vi "ziSelectDevice.vi"(3 "Error In":errorcluster, 4 "Device (first)":string, 5 "Handle In":T1 {"Handle" format="0x%08x"; "Conn" format="0x%08x"}) -> (0 "Error Out":errorcluster, 1 "Selected Device":string, 2 "Handle Out":T1 {"Handle" format="0x%08x"; "Conn" format="0x%08x"})   [LabVIEW 2016, in "Zurich Instruments LabOne.lvlib"]
doc: "Selects to the default device to use."
uses:
  Zurich Instruments LabOne.lvlib
  ziTypeHandle.ctl
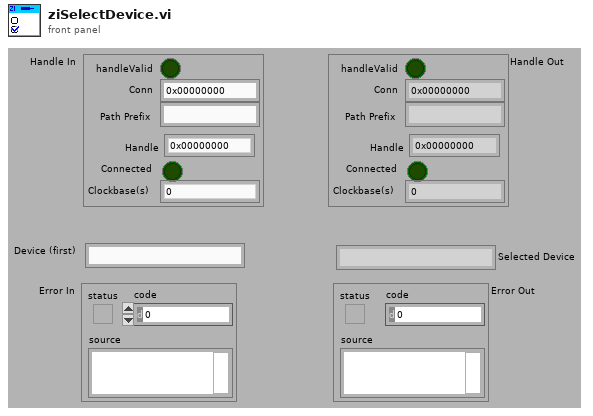
[diagram p1: front panel]
types:
  T1 = typedef "Zurich Instruments LabOne.lvlib/ziTypeHandle.ctl" = cluster{"handleValid":bool, "Conn":u64, "Path Prefix":string, "Handle":u64, "Connected":bool, "Clockbase(s)":dbl}
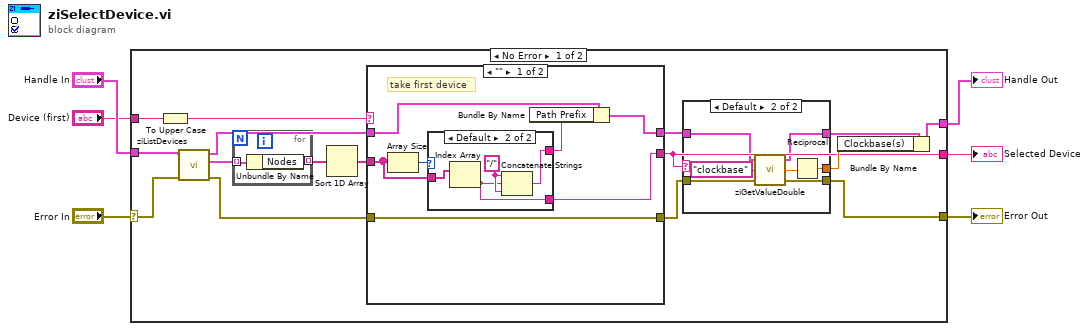
[diagram p0: block diagram]
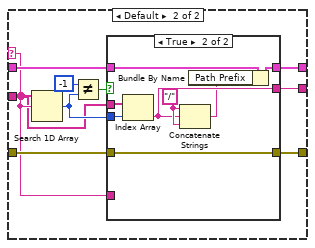
[diagram p4: hidden frame]
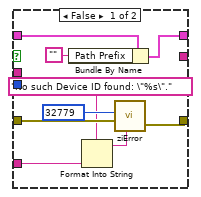
[diagram p5: hidden frame]
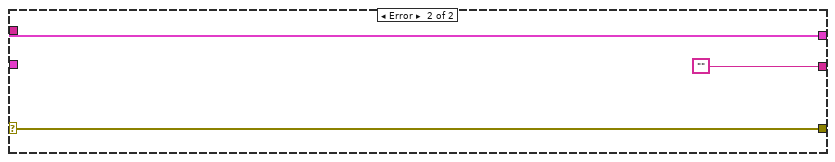
[diagram p6: hidden frame]
diagram:
  n1 = case shown="No Error" "Error In" {
    selector: "Error In" -> [w14 w72]
    tunnel: "Handle In" -> [w22 w74]
    tunnel: "Device (first)" -> [w21 _]
    tunnel: [w16 w74] -> w4
    tunnel: [w18 w72] -> w3
    tunnel: [w9 ""] -> w2
    frame No Error {
      n2 = To Upper Case(1:w21) -> (0:w13:string)
      n3 = call "ziListDevices.vi"("Error In"=w14, "Handle In"=w22) -> ("Error Out"=w12:errorcluster, "Devices"=w20:cluster{"Nodes":string, i32}[], "Handle Out"=w10:T1)  [unwired: 3 out]
      n4 = for {
        tunnel: w20 -> [w33] mode=indexing
        tunnel: [w32] -> w19 mode=indexing
        n5 = Unbundle By Name(w33) -> ("Nodes"=w32:string)
      }
      n6 = Sort 1D Array(array=w19) -> (sorted array=w7:string[])
      n7 = case shown="\"\"" w13 {
        selector: w13 -> [_ w50]
        tunnel: w7 -> [w35 w48]
        tunnel: w12 -> [w34 w51]
        tunnel: [w38 w53] -> w11
        tunnel: w10 -> [w39 w52]
        tunnel: [w36 w46] -> w9
        tunnel: [w34 w45] -> w8
        frame "" {
          # "take first device"
          n8 = Array Size(array=w35) -> (size(s)=w40:i32)
          n9 = case shown="Default" w40 {
            tunnel: [_ w43] -> w37
            tunnel: [_ w42] -> w36
            tunnel: w35 -> [_ w41]
            frame 0 {
              # "no device found"
            }
            frame Default {
              w44 = "/" ("string")
              n10 = Index Array(array=w41) -> (element=w42:string)  [unwired: 1 in]
              n11 = Concatenate Strings(w44, w42, w44) -> (w43:string)
            }
          }
          n12 = Bundle By Name(cluster=w39, "Path Prefix"=w37) -> (w38:T1)
        }
        frame Default {
          n13 = Search 1D Array(1D array=w48, element=w50) -> (index of element=w49:i32)  [unwired: 1 out]
          n14 = Not Equal?(x=-1, y=w49) -> (x != y?=w47:bool)
          n15 = case shown="True" w47 {
            tunnel: w49 -> [_ w70]
            tunnel: w48 -> [_ w71]
            tunnel: w52 -> [w63 w69]
            tunnel: [w62 w67] -> w53
            tunnel: [_ w66] -> w46
            tunnel: [w60 w64] -> w45
            tunnel: w51 -> [w61 w64]
            tunnel: w50 -> [w57 _]
            frame False {
              n16 = Bundle By Name(cluster=w63, "Path Prefix"="") -> (w62:T1)
              n17 = Format Into String(format string="No such Device ID found: \"%s\"." ("source"), w57) -> (resulting string=w56:string)  [unwired: 2 in, 1 out]
              n18 = call "ziError.vi"("ziErrorCode"=u32 32779, "Error In"=w61, "Annotation"=w56) -> ("Error Out"=w60:errorcluster)  [unwired: 3 in]
            }
            frame True {
              w68 = "/" ("string")
              n19 = Index Array(array=w71, index=w70) -> (element=w66:string)
              n20 = Concatenate Strings(w68, w66, w68) -> (w65:string)
              n21 = Bundle By Name(cluster=w69, "Path Prefix"=w65) -> (w67:T1)
            }
          }
        }
      }
      n22 = case shown="Default" w9 {
        tunnel: w11 -> [w24 w31]
        tunnel: w8 -> [w23 w29]
        tunnel: [w23 w28] -> w18
        tunnel: [w24 w27] -> w17
        tunnel: [_ w25] -> w15
        frame "" {
        }
        frame Default {
          n23 = call "ziGetValueDouble.vi"("error in"=w29, "Path"="clockbase", "Handle in"=w31) -> ("error out"=w28:errorcluster, "Value"=w26:dbl, "Handle out"=w27:T1)
          n24 = Reciprocal(x=w26) -> (1/x=w25:dbl)
        }
      }
      n25 = Bundle By Name(cluster=w17, "Clockbase(s)"=w15) -> (w16:T1)
    }
    frame Error {
    }
  }
  "Handle Out" <- w4
  "Error Out" <- w3
  "Selected Device" <- w2
